vi "tests-db.vi"() -> ()   [LabVIEW 2013]
uses:
  <vilib>/addons/database/Auxilliary.llb/DB Tools DataTypes.ctl
  <vilib>/addons/database/Connection.llb/DB Tools Open Connec (String).vi
  <vilib>/addons/database/Connection.llb/Conn Execute.vi
  <vilib>/addons/database/Recordset.llb/Rec Fetch Recordset Data (R).vi
  <vilib>/addons/database/Recordset.llb/Rec Destroy - Connection.vi
  <vilib>/addons/database/_DB Variant To Data/Database Variant To Data.xnode
  <vilib>/addons/database/NI_Database_API.lvlib
  <vilib>/addons/database/Recordset.llb/Rec Fetch Integer Data (R).vi
  2013/447 Gotec - Bancs Test G01/Automation/Labview/Local Labview_actuel/ADS.llb/Global DIOs.vi
panel:
  in  "Listbox":i32(listbox)
  out "subarray":string[](array[string])
  out "data 2":string[][](array[string])
  in  "string 2":string
  out "recordset data":variant[][](array[variant])
  out "columns":string[](array[string])
  out "column information":T2(array[cluster])
  in  "stop":bool
  out "data":variant[][](array[variant])
  out "tables":string[](array[string])
  out "Nbre de lignes":i32
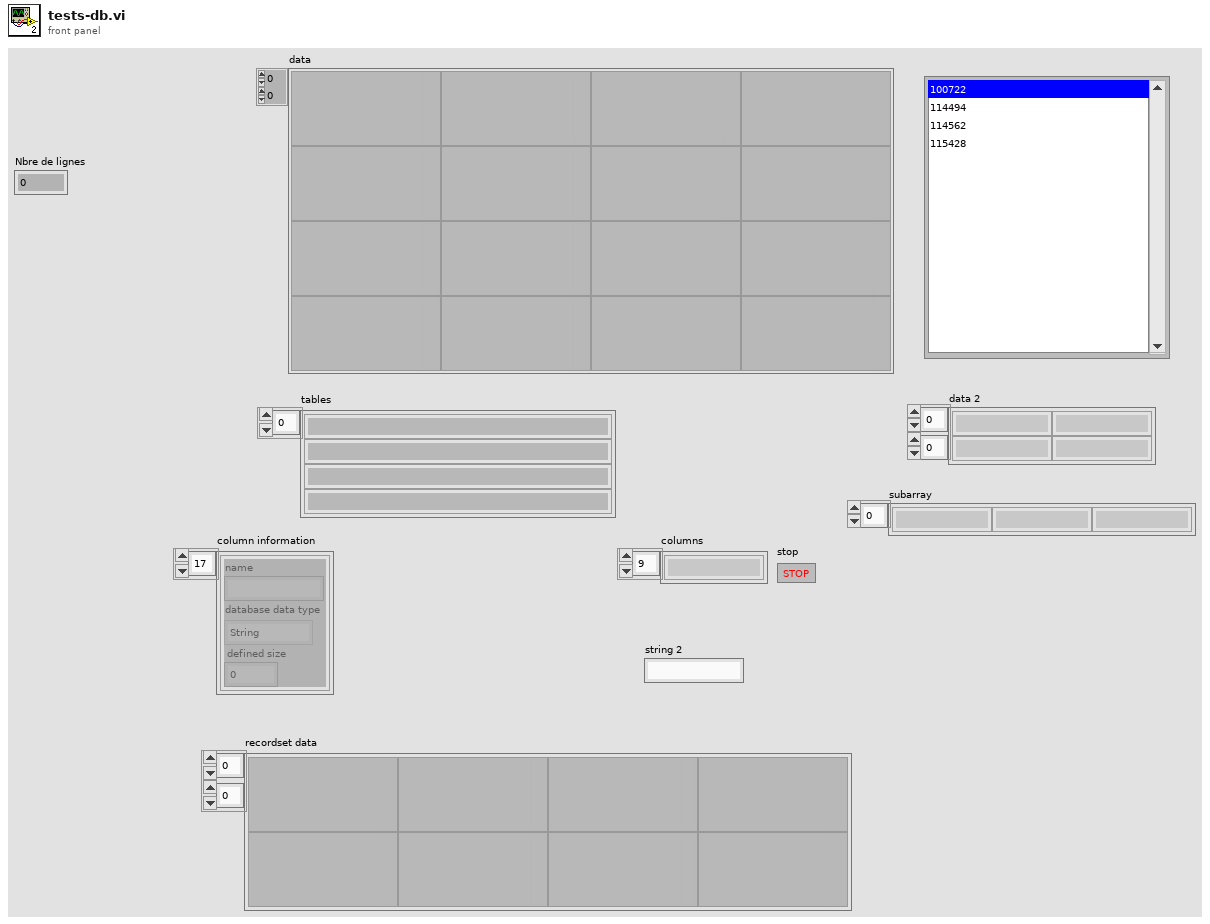
[diagram p1: front panel]
types:
  T1 = typedef "NI_Database_API.lvlib/DB Tools DataTypes.ctl" = enum16{"String", "Long (I32)", "Single (SGL)", "Double (DBL)", "Date/Time", "Binary"}
  T2 = cluster{"name":string, "database data type":T1, "defined size":i32}[]
  T3 = typedef "NI_Database_API.lvlib/Conn ObjectReference.ctl" = refnum<k1>
  T4 = cluster{"Date / Heure":string, "No Machine":string, "Type produit":u16, "Temps de chauffe":sgl, "Temps de coulage":sgl, "Temps total":sgl, "Volume en tasse":sgl, "Temperature extraction":sgl, "Courant max":sgl, "Status":u16}
  T5 = typedef "NI_Database_API.lvlib/Rec ObjectReference.ctl" = refnum<k1>
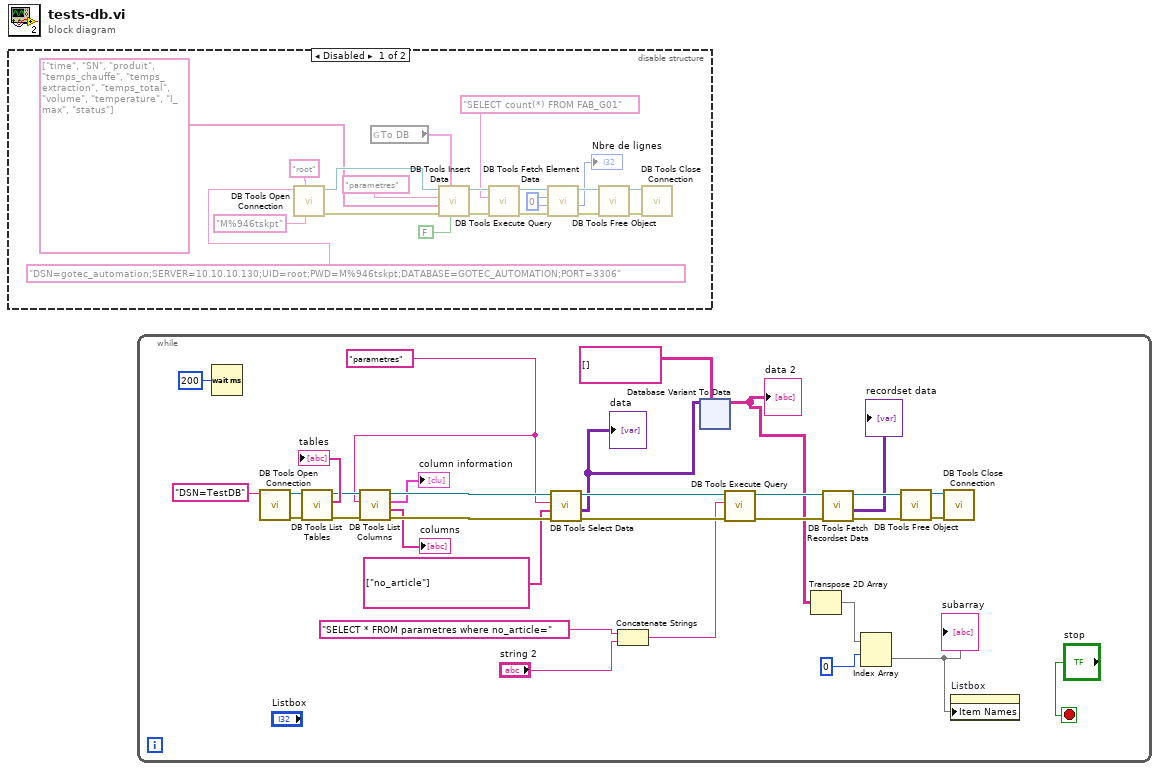
[diagram p0: block diagram]
diagram:
  n1 = disable-structure shown="Disabled" {
    frame Disabled {
      w5 = 0
      n2 = call-poly <vilib>:"DB Tools Open Connection.vi"("password"="M%946tskpt", "userID"="root", "connection information"="DSN=gotec_automation;SERVER=10.10.10.130;UID=root;PWD=M%946tskpt;DATABASE=GOTEC_AUTOMATION;PORT=3306") -> ("error out"=w17:errorcluster, "connection reference"=w18:T3)  [unwired: 5 in]
      n3 = global read "Global DIOs.vi" "To DB"() -> (w1:T4)
      n4 = call <vilib>:"DB Tools Insert Data.vi"("flatten cluster? (F)"=FALSE, "data"=w1, "error in (no error)"=w17, "columns"=string[] ["time", "SN", "produit", "temps_chauffe", "temps_extraction", "temps_total", "volume", "temperature", "I_max", "status"], "table"="parametres", "connection reference"=w18) -> ("error out"=w8:errorcluster, "connection reference out"=w9:T3)  [unwired: 4 in]
      n5 = call-poly <vilib>:"DB Tools Execute Query.vi"("error in (no error)"=w8, "SQL query"="SELECT count(*) FROM FAB_G01", "connection reference"=w9) -> ("error out"=w14:errorcluster, "recordset reference"=w10:T5)  [unwired: 5 in]
      n6 = call-poly <vilib>:"DB Tools Fetch Element Data.vi"("error in (no error)"=w14, "type"=w5, "column index"=w5, "recordset reference"=w10) -> ("error out"=w13:errorcluster, "data"=→"Nbre de lignes":i32, "recordset reference out"=w11:T5)  [unwired: 3 in]
      n7 = call-poly <vilib>:"DB Tools Free Object.vi"("error in (no error)"=w13, "recordset reference"=w11) -> ("error out"=w7:errorcluster, "connection reference"=w12:T3)  [unwired: 8 in]
      n8 = call <vilib>:"DB Tools Close Connection.vi"("error in (no error)"=w7, "connection reference"=w12) -> ()  [unwired: 5 in, 1 out]
    }
    frame Enabled {
    }
  }
  n9 = while {
    stop <- "stop" stop-if-true
    w42 = "parametres" ("table")
    n10 = Wait (ms)(milliseconds to wait=u32 200) -> ()  [unwired: 1 out]
    n11 = call-poly <vilib>:"DB Tools Open Connection.vi"("connection information"="DSN=TestDB") -> ("error out"=w51:errorcluster, "connection reference"=w50:T3)  [unwired: 7 in]
    n12 = call <vilib>:"DB Tools List Tables.vi"("error in (no error)"=w51, "connection reference"=w50) -> ("error out"=w44:errorcluster, "tables"=→"tables":string[], "connection reference out"=w46:T3)  [unwired: 3 in]
    n13 = call <vilib>:"DB Tools List Columns.vi"("error in (no error)"=w44, "table"=w42, "connection reference"=w46) -> ("error out"=w43:errorcluster, "columns"=→"columns":string[], "column information"=→"column information":T2, "connection reference out"=w45:T3)  [unwired: 1 in]
    n14 = call <vilib>:"DB Tools Select Data.vi"("error in (no error)"=w43, "columns"=string[] ["no_article"], "table"=w42, "connection reference"=w45) -> ("error out"=w39:errorcluster, "data"=w25:variant[][], "connection reference out"=w38:T3)  [unwired: 2 in]
    "data" <- w25
    n15 = Concatenate Strings("SELECT * FROM parametres where no_article=" ("SQL query"), "string 2") -> (w28:string)
    n16 = xnode "Database Variant To Data"("database variant"=w25, "type"=string[][] []) -> ("data"=w24:string[][])  [unwired: 1 in, 1 out]
    "data 2" <- w24
    n17 = call-poly <vilib>:"DB Tools Execute Query.vi"("error in (no error)"=w39, "SQL query"=w28, "connection reference"=w38) -> ("error out"=w32:errorcluster, "recordset reference"=w34:T5)  [unwired: 5 in]
    n18 = Transpose 2D Array(2D array=w24) -> (transposed array=w23:string[][])
    n19 = call-poly <vilib>:"DB Tools Fetch Recordset Data.vi"("error in (no error)"=w32, "recordset reference"=w34) -> ("error out"=w31:errorcluster, "recordset data"=→"recordset data":variant[][], "recordset reference out"=w33:T5)  [unwired: 3 in]
    n20 = Index Array(array=w23, index (row)=0 ("index")) -> (element=w21:string[])  [unwired: 1 in]
    "subarray" <- w21
    n21 = call-poly <vilib>:"DB Tools Free Object.vi"("error in (no error)"=w31, "recordset reference"=w33) -> ("error out"=w36:errorcluster, "connection reference"=w37:T3)  [unwired: 8 in]
    n22 = call <vilib>:"DB Tools Close Connection.vi"("error in (no error)"=w36, "connection reference"=w37) -> ()  [unwired: 5 in, 1 out]
    n23 = property on="Listbox" class="LstBox (strict)"("Item Names"=w21) -> ()  [unwired: 2 in, 2 out]
  }
